vi "SR_Nand.vi"() -> ()   [LabVIEW 2023]
panel:
  in  "stop":bool
  in  "CLK":bool
  in  "RESET":bool
  in  "SET":bool
  out "Q":bool
  out "Q'":bool
  # "Tablica Stanów\n\nR \tS \t   Q  Q'\nL \tL    \t Q  Q'       \nH\tL    \t H L       \t \nL \tH    \tL  L    \t\nH \tH    X  X"
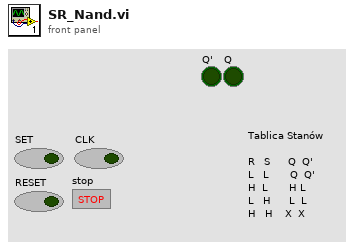
[diagram p1: front panel]
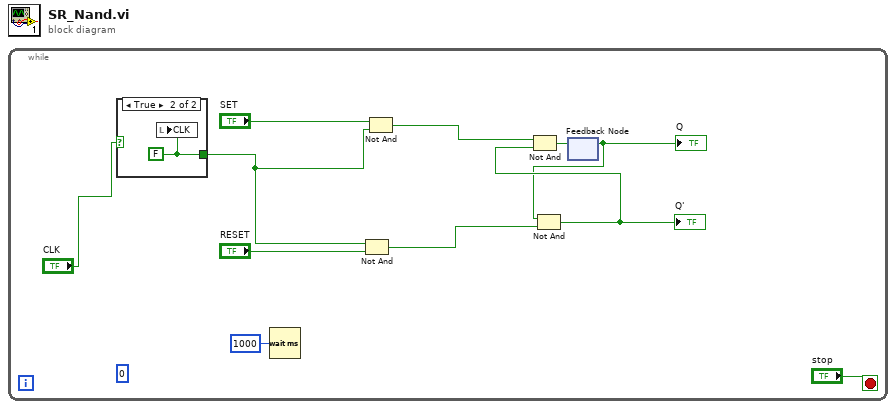
[diagram p0: block diagram]
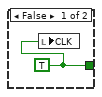
[diagram p2: hidden frame]
diagram:
  n1 = while {
    stop <- "stop" stop-if-true
    (unwired) 0
    n2 = case shown="True" "CLK" {
      tunnel: [w12 w13] -> w6
      frame False {
        w12 = TRUE
        n3 = local write "CLK"(w12) -> ()
      }
      frame True {
        w13 = FALSE
        n4 = local write "CLK"(w13) -> ()
      }
    }
    n5 = Wait (ms)(milliseconds to wait=u32 1000) -> ()  [unwired: 1 out]
    n6 = Not And(1:"RESET", 2:w6) -> (0:w8:bool)
    n7 = Not And(1:w6, 2:"SET") -> (0:w7:bool)
    n8 = feedback #1() -> (w1:bool)  [unwired: 1 in]
    "Q" <- w1
    n9 = Not And(1:w8, 2:w1) -> (0:w3:bool)
    "Q'" <- w3
    n10 = Not And(1:w3, 2:w7) -> (0:w2:bool)
    n11 = feedback-in #1(w2) -> ()
  }
